vi "MarkSelected.vi"(0 "MapPositions":refnum<vi>, 1 "PadLookup":refnum<vi>, 2 "WaferPads":refnum<vi>, 3 "Id":string, 4 "Enum":enum16{"Remove", "Mark", "Clear All"}(ring), 6 "MeasureControl":refnum<vi>) -> ()   [LabVIEW 2012]
uses:
  Controls/SelectedPads.ctl
  Controls/Pad.ctl
  Controls/MeasureControl.ctl
  Controls/PadArea.ctl
  Controls/TestData.ctl
  Controls/Measurement.ctl
panel:
  # "Measure Control"
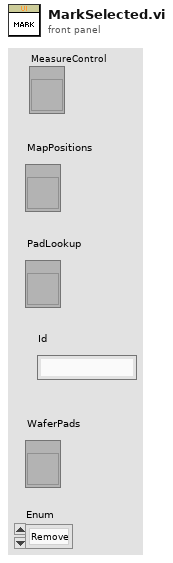
[diagram p1: front panel]
types:
  T1 = typedef "MapPOS.ctl" = cluster{"Coords":cluster{"Horizontal":sgl, "Vertical":sgl}, "radius":i32, "state":bool, "Id":string}[]
  T2 = typedef "Pad.ctl" = cluster{"Coords":cluster{"Horizontal":sgl, "Vertical":sgl}, "radius":i32, "Tested":bool, "Selected":bool, "Id":string}
  T3 = typedef "SelectedPads.ctl" = T2[]
  T4 = typedef "PadLookup.ctl" = cluster{"A":T5, "B":T5, "C":T5, "D":T5, "L":T5, "R":T5, "T":T5, "G":T5}
  T5 = typedef "PadLookupItem.ctl" = cluster{"PadArea":T6, string[]}
  T6 = typedef "PadArea.ctl" = enum16{"CenterA", "CenterB", "CenterC", "CenterD", "L", "R", "T", "G"}
  T7 = typedef "MeasureControl.ctl" = cluster{"Graph":cluster{"Y":dbl[], "Y":dbl[]}[], "Wafer Area":T6, "Pad":string, "Measure":bool, "Cluster 2":cluster{"TestData":T8, "Pass":bool, "Fail":bool}}
  T8 = typedef "TestData.ctl" = cluster{"20mA Data":T9, "50mA Data ":T9}
  T9 = typedef "Measurement.ctl" = cluster{"Area":string, "Pad":string, "Current,mA":dbl, "Power":dbl, "WL":dbl, "Voltage":dbl, "Knee Current":dbl, "Reverse":dbl}
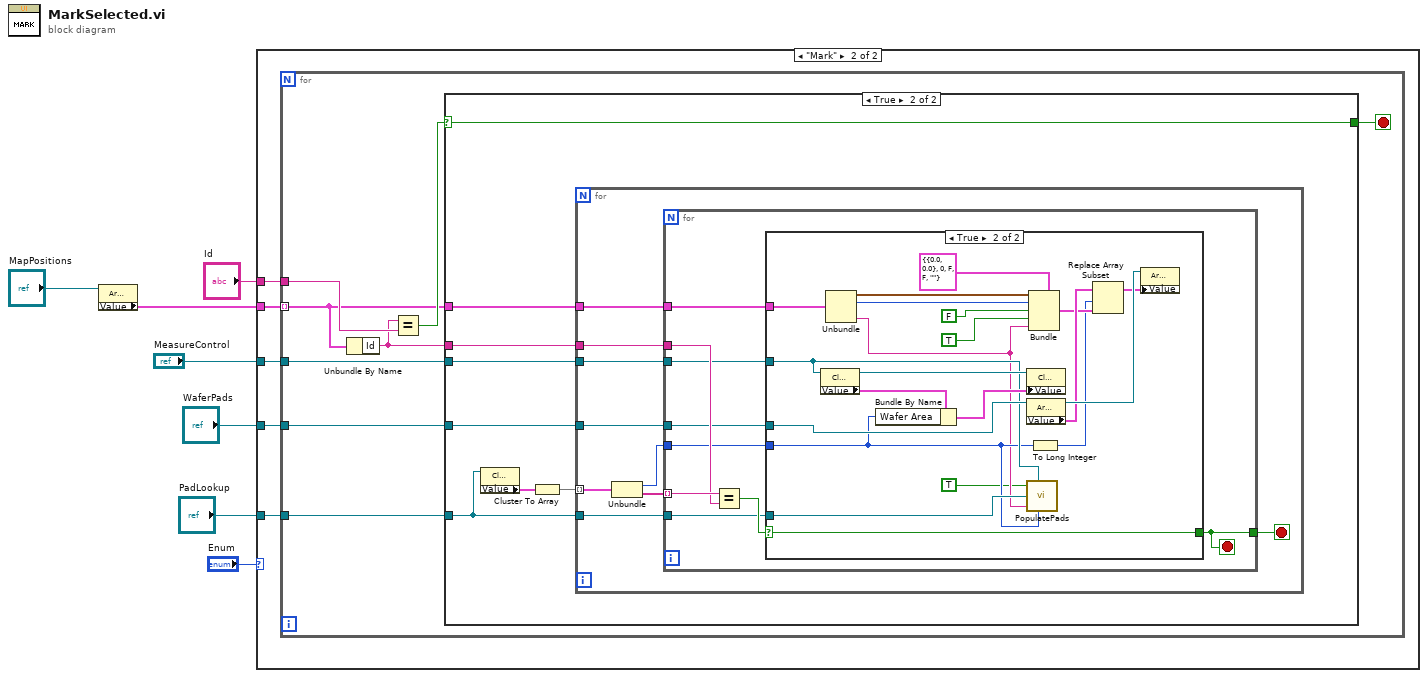
[diagram p0: block diagram]
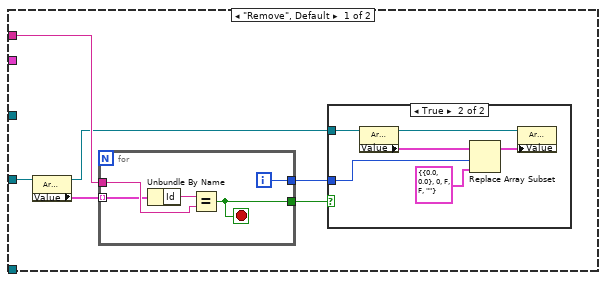
[diagram p2: hidden frame]
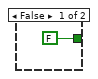
[diagram p4: hidden frame]
diagram:
  n1 = property class="Arr (strict)"(reference="MapPositions") -> ("Value"=w6:T1)  [unwired: 1 in, 2 out]
  n2 = case shown="\"Mark\"" "Enum" {
    tunnel: w6 -> [_ w29]
    tunnel: "Id" -> [w11 w28]
    tunnel: "PadLookup" -> [_ w27]
    tunnel: "WaferPads" -> [w13 w26]
    tunnel: "MeasureControl" -> [_ w25]
    frame "Remove", Default {
      n3 = property class="Arr (strict)"(reference=w13) -> (reference out=w8:refnum<vi>, "Value"=w12:T3)  [unwired: 1 in, 1 out]
      n4 = for {
        tunnel: w12 -> [w23] mode=indexing
        tunnel: w11 -> [w24]
        tunnel: [w20] -> w9
        tunnel: [w21] -> w10
        i -> [w20]
        stop <- w21 stop-if-true
        n5 = Unbundle By Name(w23) -> ("Id"=w22:string)
        n6 = Equal?(x=w22, y=w24) -> (x = y?=w21:bool)
      }
      n7 = case shown="True" w10 {
        tunnel: w9 -> [_ w16]
        tunnel: w8 -> [_ w19]
        frame False {
        }
        frame True {
          n8 = property class="Arr (strict)"(reference=w19) -> (reference out=w18:refnum<vi>, "Value"=w17:T3)  [unwired: 1 in, 1 out]
          n9 = Replace Array Subset(array=w17, new element=T2 {"Coords"={"Horizontal"=0.0, "Vertical"=0.0}, "radius"=0, "Tested"=FALSE, "Selected"=FALSE, "Id"=""} ("new element/subarray"), index=w16) -> (w14:T3)
          n10 = property class="Arr (strict)"(reference=w18, "Value"=w14) -> ()  [unwired: 1 in, 2 out]
        }
      }
    }
    frame "Mark" {
      n11 = for {
        tunnel: w29 -> [w31] mode=indexing
        tunnel: w28 -> [w37]
        tunnel: w27 -> [w34]
        tunnel: w26 -> [w32]
        tunnel: w25 -> [w30]
        stop <- w35 stop-if-true
        n12 = Unbundle By Name(w31) -> ("Id"=w33:string)
        n13 = Equal?(x=w33, y=w37) -> (x = y?=w36:bool)
        n14 = case shown="True" w36 {
          selector: w36 -> [_ w46]
          tunnel: [FALSE w46] -> w35
          tunnel: w34 -> [_ w39]
          tunnel: w33 -> [_ w43]
          tunnel: w32 -> [_ w42]
          tunnel: w31 -> [_ w41]
          tunnel: w30 -> [_ w40]
          frame False {
          }
          frame True {
            n15 = property class="Clust (strict)"(reference=w39) -> ("Value"=w45:T4)  [unwired: 1 in, 2 out]
            n16 = Cluster To Array(cluster=w45) -> (array=w44:T5[])
            n17 = for {
              tunnel: w44 -> [w51] mode=indexing
              tunnel: w43 -> [w54]
              tunnel: w42 -> [w53]
              tunnel: w41 -> [w50]
              tunnel: w40 -> [w48]
              tunnel: w39 -> [w47]
              stop <- w49 stop-if-true
              n18 = Unbundle(w51) -> ("PadArea"=w52:T6, w55:string[])
              n19 = for {
                tunnel: w55 -> [w64] mode=indexing
                tunnel: w54 -> [w63]
                tunnel: w53 -> [w61]
                tunnel: w52 -> [w60]
                tunnel: w50 -> [w59]
                tunnel: [w58] -> w49
                tunnel: w48 -> [w57]
                tunnel: w47 -> [w56]
                stop <- w58 stop-if-true
                n20 = Equal?(x=w64, y=w63) -> (x = y?=w62:bool)
                n21 = case shown="True" w62 {
                  selector: w62 -> [w65 w75]
                  tunnel: w61 -> [_ w85]
                  tunnel: w60 -> [_ w68]
                  tunnel: w59 -> [_ w81]
                  tunnel: [w65 w75] -> w58
                  tunnel: w57 -> [_ w70]
                  tunnel: w56 -> [_ w69]
                  frame False {
                  }
                  frame True {
                    n22 = property class="Clust (strict)"(reference=w70) -> (reference out=w72:refnum<vi>, "Value"=w73:T7)  [unwired: 1 in, 1 out]
                    n23 = Unbundle(w81) -> ("Coords"=w80:cluster{"Horizontal":sgl, "Vertical":sgl}, "radius"=w78:i32, "Id"=w67:string)  [unwired: 1 out]
                    n24 = Bundle By Name(cluster=w73, "Wafer Area"=w68) -> (w71:T7)
                    n25 = property class="Clust (strict)"(reference=w72, "Value"=w71) -> ()  [unwired: 1 in, 2 out]
                    n26 = property class="Arr (strict)"(reference=w85) -> (reference out=w86:refnum<vi>, "Value"=w84:T3)  [unwired: 1 in, 1 out]
                    n27 = call "PopulatePads.vi"("Set Pad?"=TRUE, "MeasureControl"=w70, "PadLookup"=w69, "Pad"=w67, "PadArea"=w68) -> ()  [unwired: 1 in]
                    n28 = Bundle(cluster=T2 {"Coords"={"Horizontal"=0.0, "Vertical"=0.0}, "radius"=0, "Tested"=FALSE, "Selected"=FALSE, "Id"=""} ("new element/subarray"), "Coords"=w80, "radius"=w78, "Tested"=FALSE, "Selected"=TRUE, "Id"=w67) -> (w77:T2)
                    n29 = To Long Integer(number=w68) -> (32bit integer=w74:i32)
                    n30 = Replace Array Subset(array=w84, new element=w77, index=w74) -> (w76:T3)
                    n31 = property class="Arr (strict)"(reference=w86, "Value"=w76) -> ()  [unwired: 1 in, 2 out]
                  }
                }
              }
            }
          }
        }
      }
    }
  }
